vi "ProyectoFinal.vi"() -> ()   [LabVIEW 2024]
uses:
  <vilib>/httpClient/PUTBuffer.vi
  <vilib>/httpClient/LabVIEWHTTPClient.lvlib
panel:
  out "error out":errorcluster
  in  "Modificar valores":bool
  out "body":string
  out "headers":string
  out "error GET 7":errorcluster {"code" format="%f"}
  out "error GET 6":errorcluster {"code" format="%f"}
  out "error GET 5":errorcluster {"code" format="%f"}
  out "error GET 4":errorcluster {"code" format="%f"}
  out "error GET 3":errorcluster {"code" format="%f"}
  out "error GET 2":errorcluster {"code" format="%f"}
  in  "Controles":T1(tab)
  out "Ki":dbl
  out "K":dbl
  out "Kd":dbl
  out "sp":dbl
  in  "Ki":dbl
  in  "Kd":dbl
  in  "K":dbl
  in  "Posicion Motor":dbl(knob) scale=0.0..360.0
  out "KI":dbl
  out "KP":dbl
  out "RPM 2":dbl
  in  "KI":dbl
  in  "RPM":dbl(knob) scale=0.0..255.0
  in  "KP":dbl
  out "Set-Point":dbl
  out "Sensor":dbl
  out "Kd":dbl
  out "dt":dbl
  out "Ki":dbl
  out "K":dbl
  in  "Set-Point":dbl(knob) scale=0.0..360.0
  in  "kd":dbl
  in  "ki":dbl
  in  "kp":dbl
  out "RPM":dbl
  out "KI":dbl
  out "KP":dbl
  in  "RPM":dbl(knob) scale=0.0..255.0
  in  "KI":dbl
  in  "KP":dbl
  out "Ki":dbl
  out "K":dbl
  out "Kd":dbl
  out "SetPoint":dbl
  out "Temp":dbl
  in  "SetPoint":dbl(slide) scale=0.0..100.0
  in  "Ki":dbl
  in  "K":dbl
  in  "Kd":dbl
  out "Boolean":bool
  in  "Secuencia":string
  in  "Aceptar":bool
  out "Secuencia":string
  out "KP":dbl
  out "KI":dbl
  out "RPM":dbl
  in  "KP":dbl
  in  "RPM":dbl(knob) scale=0.0..10.0
  in  "KI":dbl
  in  "stop":bool
  out "error GET":errorcluster {"code" format="%f"}
  out "body GET":string
  out "headers GET":string
  # "ON"
  # "OFF"
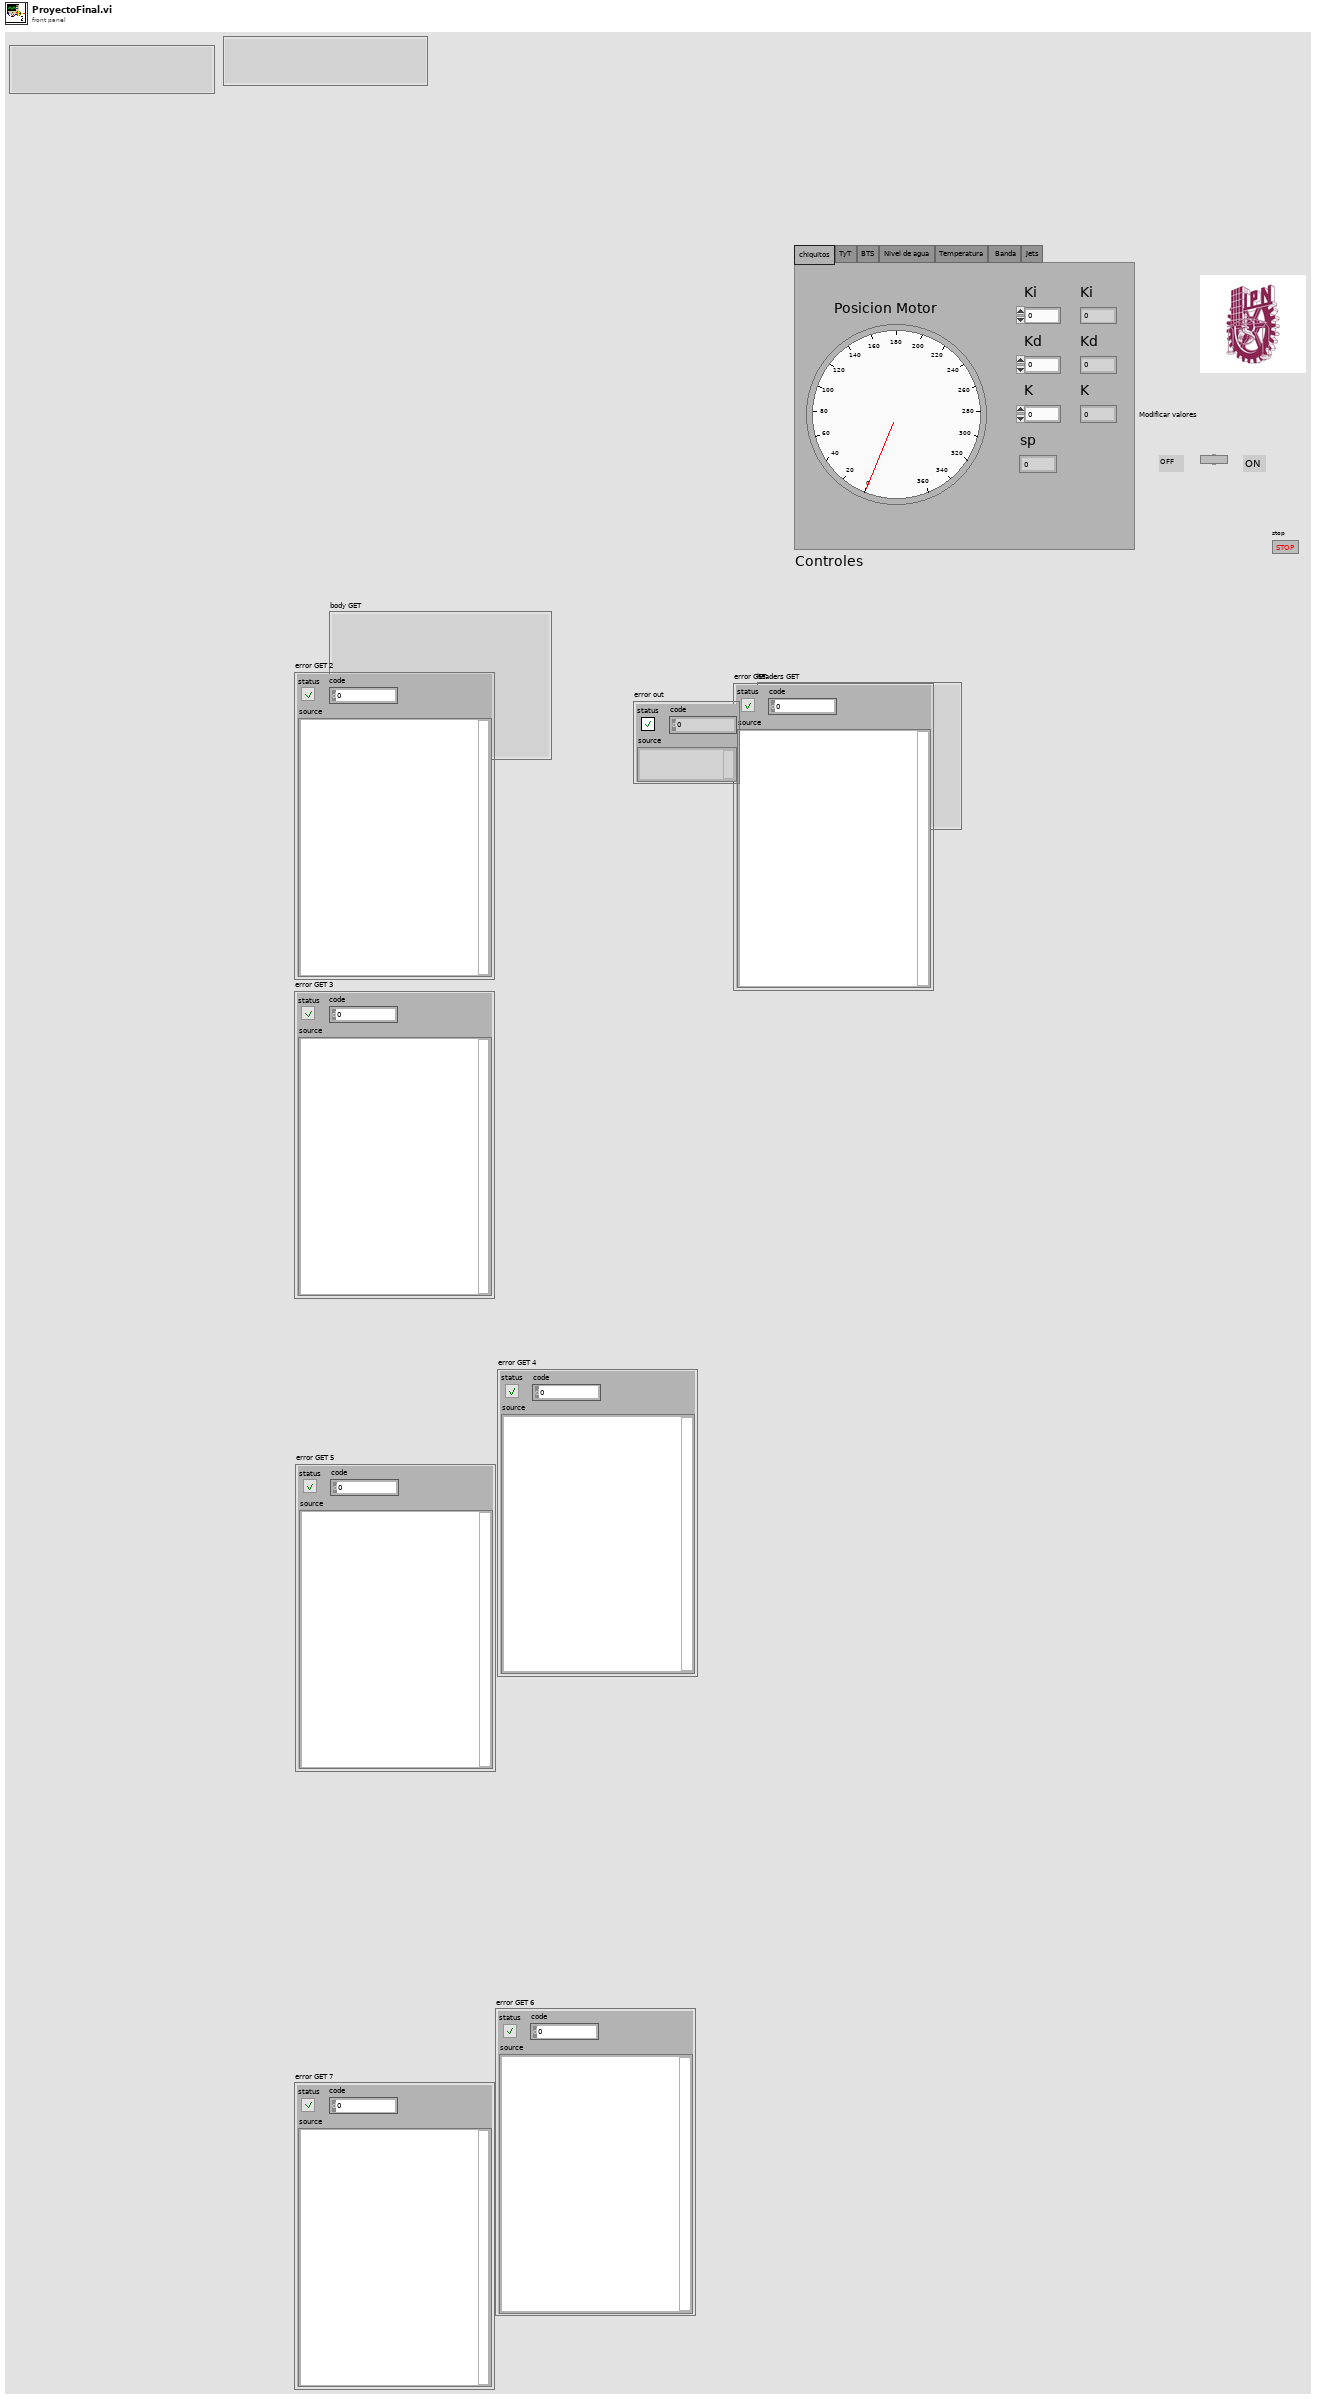
[diagram p1: front panel]
types:
  T1 = enum32{"chiquitos", "TyT", "BTS", "Nivel de agua", "Temperatura", " Banda", "Jets"}
  T2 = cluster{"Sensor":dbl, "Set-Point":dbl, "dt":dbl, "kd":dbl, "ki":dbl, "kp":dbl}
  T3 = cluster{"K":dbl, "Kd":dbl, "Ki":dbl, "SetPoint":dbl, "Temp":dbl}
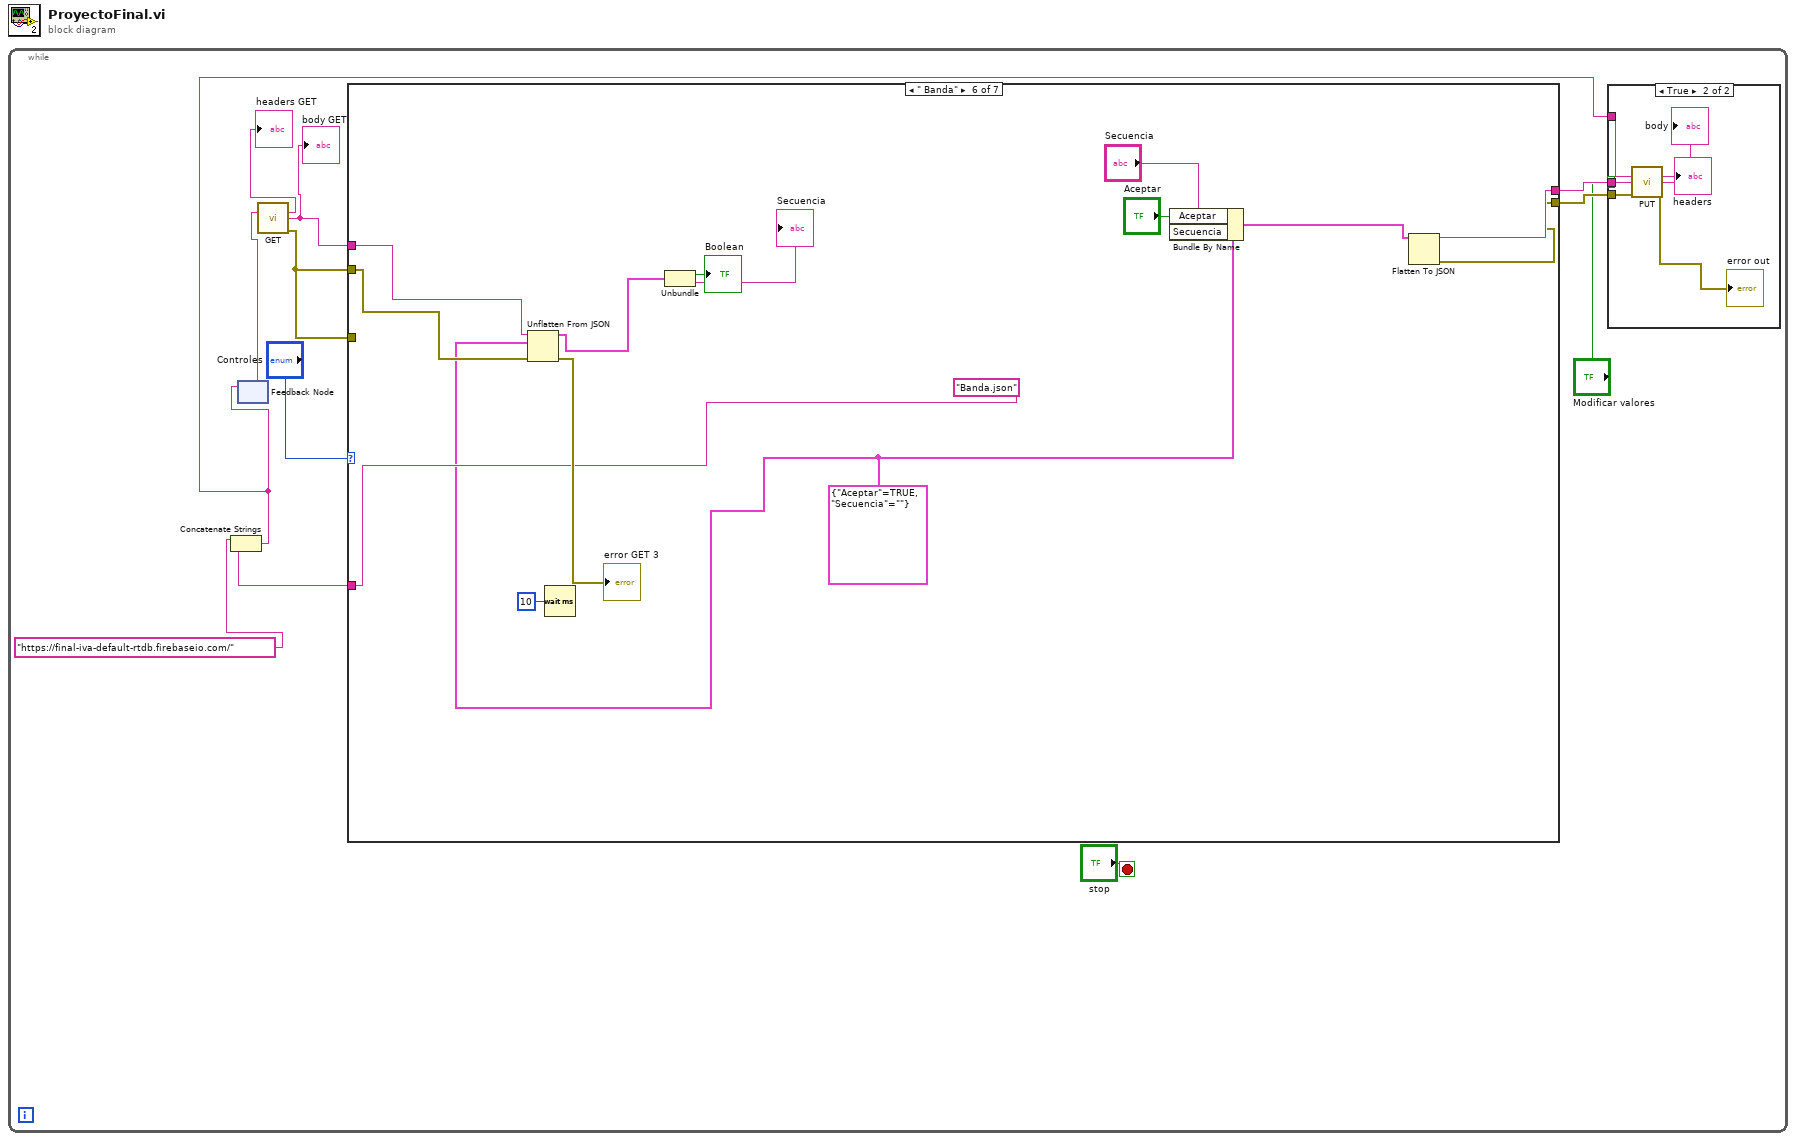
[diagram p0: block diagram]
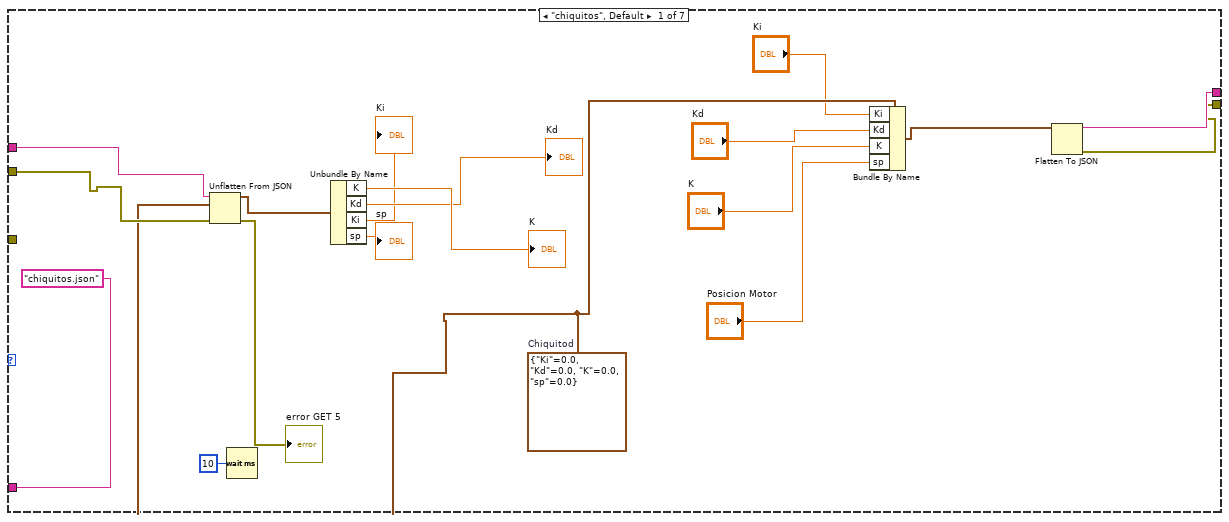
[diagram p3: hidden frame]
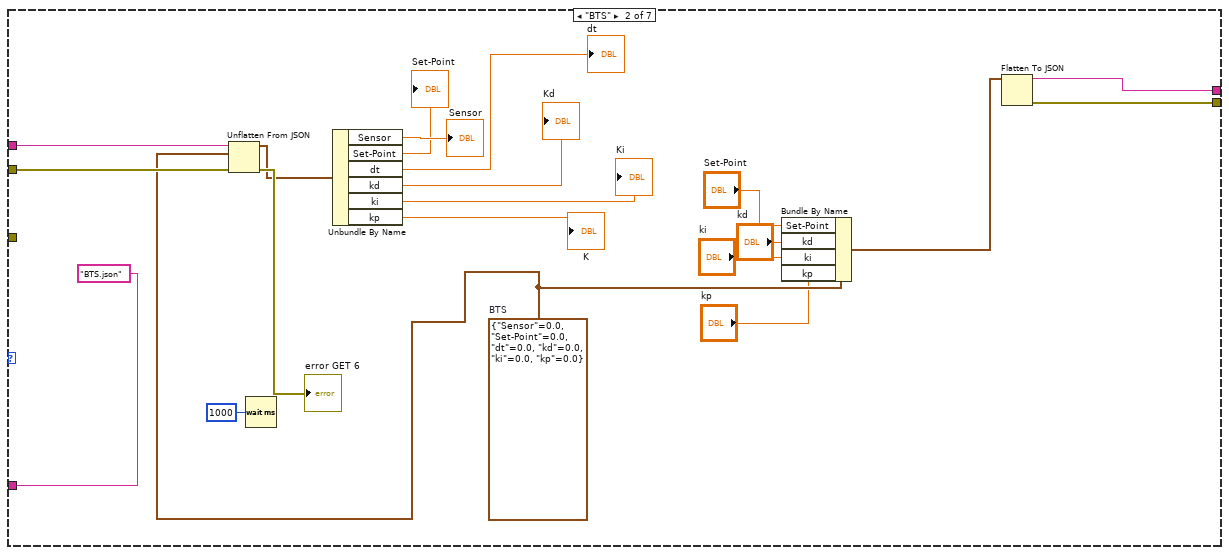
[diagram p4: hidden frame]
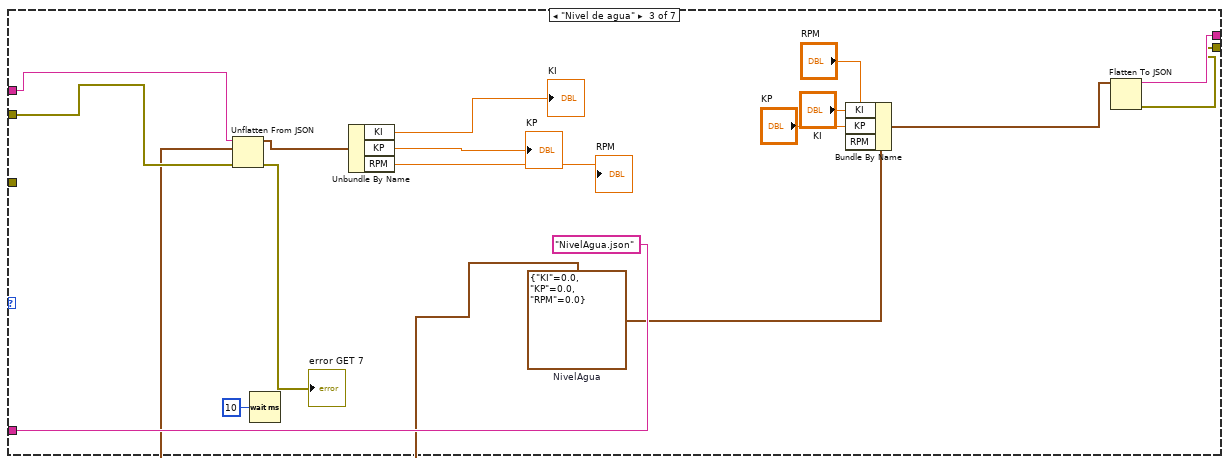
[diagram p5: hidden frame]
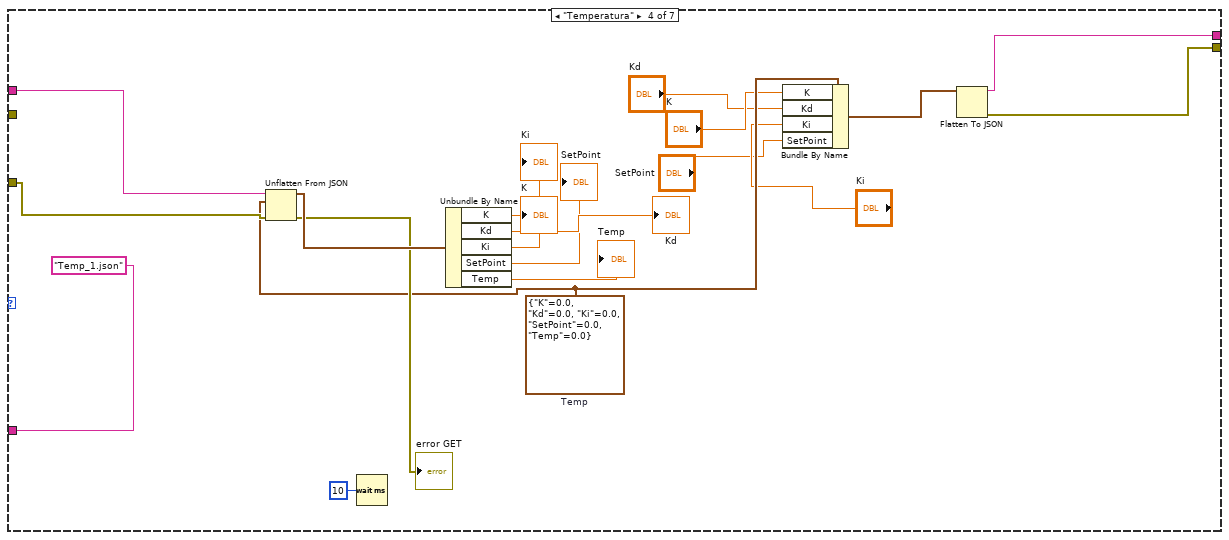
[diagram p6: hidden frame]
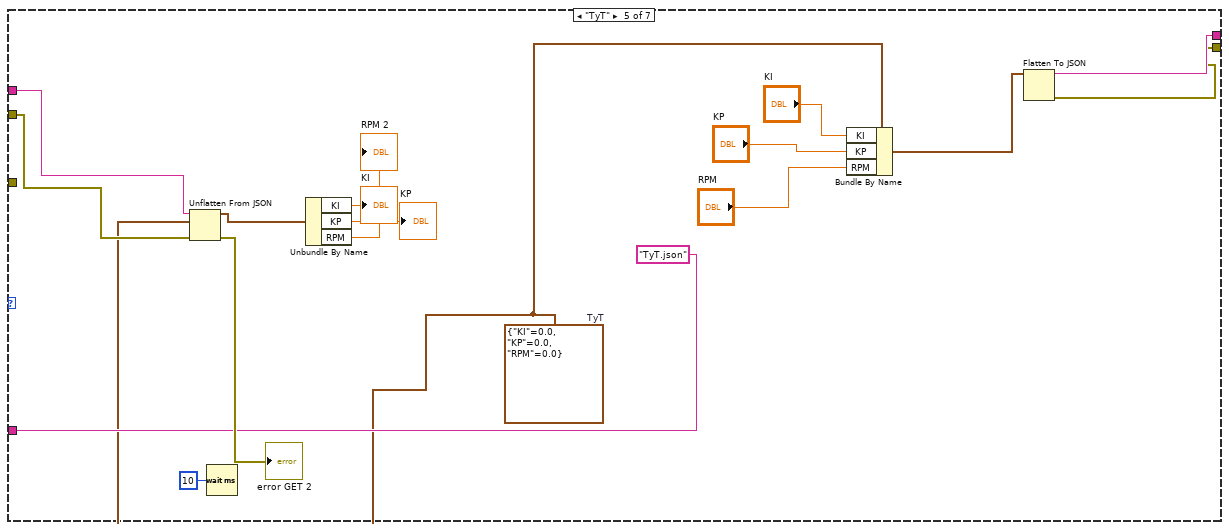
[diagram p7: hidden frame]
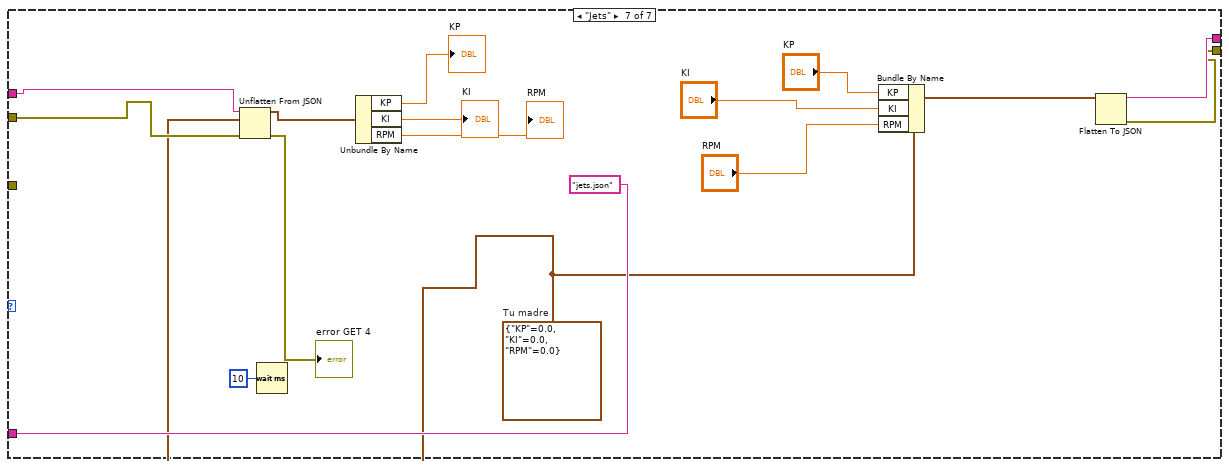
[diagram p8: hidden frame]
diagram:
  n1 = while {
    stop <- "stop" stop-if-true
    n2 = feedback #1() -> (w6:string)  [unwired: 1 in]
    n3 = call <vilib>:"GET.vi"("url"=w6) -> ("headers"=→"headers GET":string, "body"=w7:string, "error out"=w5:errorcluster)  [unwired: 11 in, 1 out]
    "body GET" <- w7
    n4 = case shown="\" Banda\"" "Controles" {
      tunnel: ["chiquitos.json" "BTS.json" "NivelAgua.json" "Temp_1.json" "TyT.json" "Banda.json" "jets.json"] -> w9
      tunnel: w7 -> [w28 w46 w64 w84 w100 w115 w130]
      tunnel: w5 -> [w27 w45 w65 _ w99 w116 w129]
      tunnel: w5 -> [_ _ _ w83 _ _ _]
      tunnel: [w24 w44 w63 w78 w96 w113 w127] -> w4
      tunnel: [w23 w43 w62 w77 w95 w112 w126] -> w3
      frame "chiquitos", Default {
        w26 = cluster{"Ki":dbl, "Kd":dbl, "K":dbl, "sp":dbl} {"Ki"=0.0, "Kd"=0.0, "K"=0.0, "sp"=0.0}  # Chiquitod
        n5 = Unflatten From JSON(JSON string=w28, type and defaults=w26, error in (no error)=w27) -> (value=w34:cluster{"Ki":dbl, "Kd":dbl, "K":dbl, "sp":dbl}, error out=→"error GET 5":errorcluster)  [unwired: 4 in]
        n6 = Wait (ms)(milliseconds to wait=u32 10) -> ()  [unwired: 1 out]
        n7 = Unbundle By Name(w34) -> ("K"=→"K":dbl, "Kd"=→"Kd":dbl, "Ki"=→"Ki":dbl, "sp"=→"sp":dbl)
        n8 = Bundle By Name(cluster=w26, "Ki"="Ki", "Kd"="Kd", "K"="K", "sp"="Posicion Motor") -> (w25:cluster{"Ki":dbl, "Kd":dbl, "K":dbl, "sp":dbl})
        n9 = Flatten To JSON(anything=w25) -> (JSON string=w24:string, 11:w23:errorcluster)  [unwired: 2 in]
      }
      frame "BTS" {
        w42 = T2 {"Sensor"=0.0, "Set-Point"=0.0, "dt"=0.0, "kd"=0.0, "ki"=0.0, "kp"=0.0}  # BTS
        n10 = Unflatten From JSON(JSON string=w46, type and defaults=w42, error in (no error)=w45) -> (value=w54:T2, error out=→"error GET 6":errorcluster)  [unwired: 4 in]
        n11 = Wait (ms)(milliseconds to wait=u32 1000) -> ()  [unwired: 1 out]
        n12 = Unbundle By Name(w54) -> ("Sensor"=→"Sensor":dbl, "Set-Point"=→"Set-Point":dbl, "dt"=→"dt":dbl, "kd"=→"Kd":dbl, "ki"=→"Ki":dbl, "kp"=→"K":dbl)
        n13 = Bundle By Name(cluster=w42, "Set-Point"="Set-Point", "kd"="kd", "ki"="ki", "kp"="kp") -> (w41:T2)
        n14 = Flatten To JSON(anything=w41) -> (JSON string=w44:string, 11:w43:errorcluster)  [unwired: 2 in]
      }
      frame "Nivel de agua" {
        w60 = cluster{"KI":dbl, "KP":dbl, "RPM":dbl} {"KI"=0.0, "KP"=0.0, "RPM"=0.0}  # NivelAgua
        n15 = Unflatten From JSON(JSON string=w64, type and defaults=w60, error in (no error)=w65) -> (value=w70:cluster{"KI":dbl, "KP":dbl, "RPM":dbl}, error out=→"error GET 7":errorcluster)  [unwired: 4 in]
        n16 = Wait (ms)(milliseconds to wait=u32 10) -> ()  [unwired: 1 out]
        n17 = Unbundle By Name(w70) -> ("KI"=→"KI":dbl, "KP"=→"KP":dbl, "RPM"=→"RPM":dbl)
        n18 = Bundle By Name(cluster=w60, "KI"="KI", "KP"="KP", "RPM"="RPM") -> (w61:cluster{"KI":dbl, "KP":dbl, "RPM":dbl})
        n19 = Flatten To JSON(anything=w61) -> (JSON string=w63:string, 11:w62:errorcluster)  [unwired: 2 in]
      }
      frame "Temperatura" {
        w80 = T3 {"K"=0.0, "Kd"=0.0, "Ki"=0.0, "SetPoint"=0.0, "Temp"=0.0}  # Temp
        n20 = Unflatten From JSON(JSON string=w84, type and defaults=w80, error in (no error)=w83) -> (value=w82:T3, error out=→"error GET":errorcluster)  [unwired: 4 in]
        n21 = Wait (ms)(milliseconds to wait=u32 10) -> ()  [unwired: 1 out]
        n22 = Unbundle By Name(w82) -> ("K"=→"K":dbl, "Kd"=→"Kd":dbl, "Ki"=→"Ki":dbl, "SetPoint"=→"SetPoint":dbl, "Temp"=→"Temp":dbl)
        n23 = Bundle By Name(cluster=w80, "K"="K", "Kd"="Kd", "Ki"="Ki", "SetPoint"="SetPoint") -> (w79:T3)
        n24 = Flatten To JSON(anything=w79) -> (JSON string=w78:string, 11:w77:errorcluster)  [unwired: 2 in]
      }
      frame "TyT" {
        w98 = cluster{"KI":dbl, "KP":dbl, "RPM":dbl} {"KI"=0.0, "KP"=0.0, "RPM"=0.0}  # TyT
        n25 = Unflatten From JSON(JSON string=w100, type and defaults=w98, error in (no error)=w99) -> (value=w105:cluster{"KI":dbl, "KP":dbl, "RPM":dbl}, error out=→"error GET 2":errorcluster)  [unwired: 4 in]
        n26 = Wait (ms)(milliseconds to wait=u32 10) -> ()  [unwired: 1 out]
        n27 = Unbundle By Name(w105) -> ("KI"=→"KI":dbl, "KP"=→"KP":dbl, "RPM"=→"RPM 2":dbl)
        n28 = Bundle By Name(cluster=w98, "KI"="KI", "KP"="KP", "RPM"="RPM") -> (w97:cluster{"KI":dbl, "KP":dbl, "RPM":dbl})
        n29 = Flatten To JSON(anything=w97) -> (JSON string=w96:string, 11:w95:errorcluster)  [unwired: 2 in]
      }
      frame " Banda" {
        w110 = cluster{"Aceptar":bool, "Secuencia":string} {"Aceptar"=TRUE, "Secuencia"=""}
        n30 = Unflatten From JSON(JSON string=w115, type and defaults=w110, error in (no error)=w116) -> (value=w118:cluster{"Aceptar":bool, "Secuencia":string}, error out=→"error GET 3":errorcluster)  [unwired: 4 in]
        n31 = Wait (ms)(milliseconds to wait=u32 10) -> ()  [unwired: 1 out]
        n32 = Unbundle(w118) -> ("Aceptar"=→"Boolean":bool, "Secuencia"=→"Secuencia":string)
        n33 = Bundle By Name(cluster=w110, "Aceptar"="Aceptar", "Secuencia"="Secuencia") -> (w114:cluster{"Aceptar":bool, "Secuencia":string})
        n34 = Flatten To JSON(anything=w114) -> (JSON string=w113:string, 11:w112:errorcluster)  [unwired: 2 in]
      }
      frame "Jets" {
        w125 = cluster{"KP":dbl, "KI":dbl, "RPM":dbl} {"KP"=0.0, "KI"=0.0, "RPM"=0.0}  # Tu madre
        n35 = Unflatten From JSON(JSON string=w130, type and defaults=w125, error in (no error)=w129) -> (value=w135:cluster{"KP":dbl, "KI":dbl, "RPM":dbl}, error out=→"error GET 4":errorcluster)  [unwired: 4 in]
        n36 = Wait (ms)(milliseconds to wait=u32 10) -> ()  [unwired: 1 out]
        n37 = Unbundle By Name(w135) -> ("KP"=→"KP":dbl, "KI"=→"KI":dbl, "RPM"=→"RPM":dbl)
        n38 = Bundle By Name(cluster=w125, "KP"="KP", "KI"="KI", "RPM"="RPM") -> (w128:cluster{"KP":dbl, "KI":dbl, "RPM":dbl})
        n39 = Flatten To JSON(anything=w128) -> (JSON string=w127:string, 11:w126:errorcluster)  [unwired: 2 in]
      }
    }
    n40 = Concatenate Strings "Concatenate Strings"("https://final-iva-default-rtdb.firebaseio.com/", w9) -> (w2:string)
    n41 = feedback-in #1(w2) -> ()
    n42 = case shown="True" "Modificar valores" {
      tunnel: w4 -> [_ w18]
      tunnel: w3 -> [_ w17]
      tunnel: w2 -> [_ w16]
      frame False {
      }
      frame True {
        n43 = call-poly <vilib>:"PUT.vi"("url"=w16, "buffer"=w18, "error in (no error)"=w17) -> ("headers"=→"headers":string, "body"=→"body":string, "error out"=→"error out":errorcluster)  [unwired: 9 in, 1 out]
      }
    }
  }
